vi "butterworth_comparison.vi"() -> ()   [LabVIEW 2022 SP3]
uses:
  <vilib>/express/express analysis/Spectral/Block/exnSpectralBlock spectral measurements peak poly.vi
  <vilib>/express/express analysis/Spectral/Block/exnSpectralBlock spectral measurements peak DDT.vi
  <vilib>/express/express analysis/Spectral/XNode/ExpressSpectralMeasurementsBlockNode.xnode
panel:
  out "Waveform Graph 4":dbl[][](graph)
  out "Waveform Graph 3":dbl[][](graph)
  out "Waveform Graph 2":dynamicdata(graph)
  out "Waveform Graph":dynamicdata(graph)
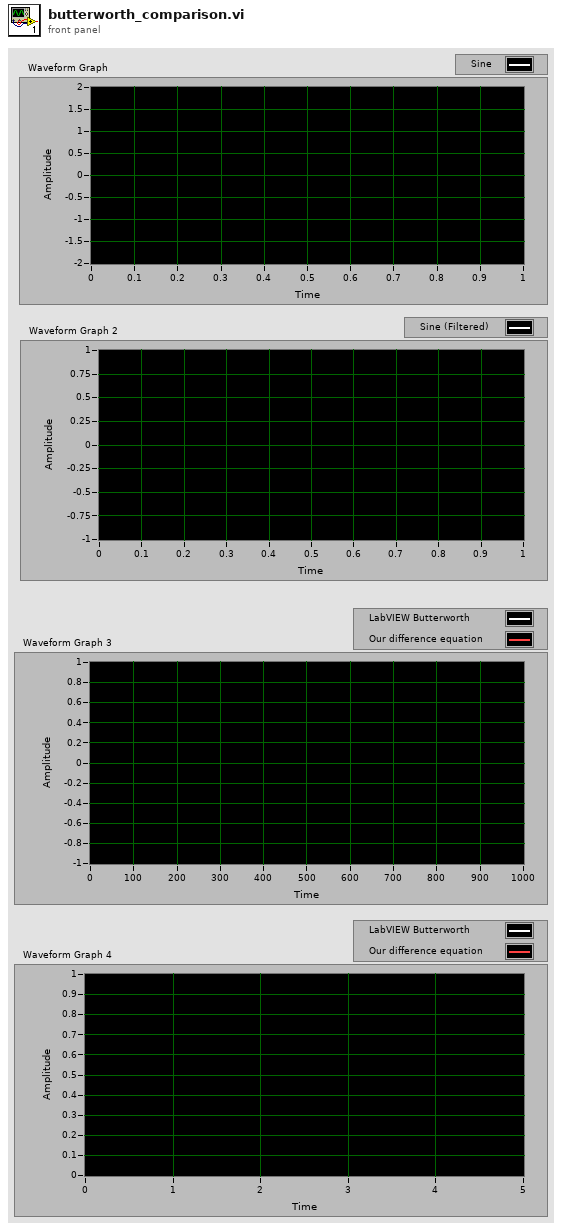
[diagram p1: front panel]
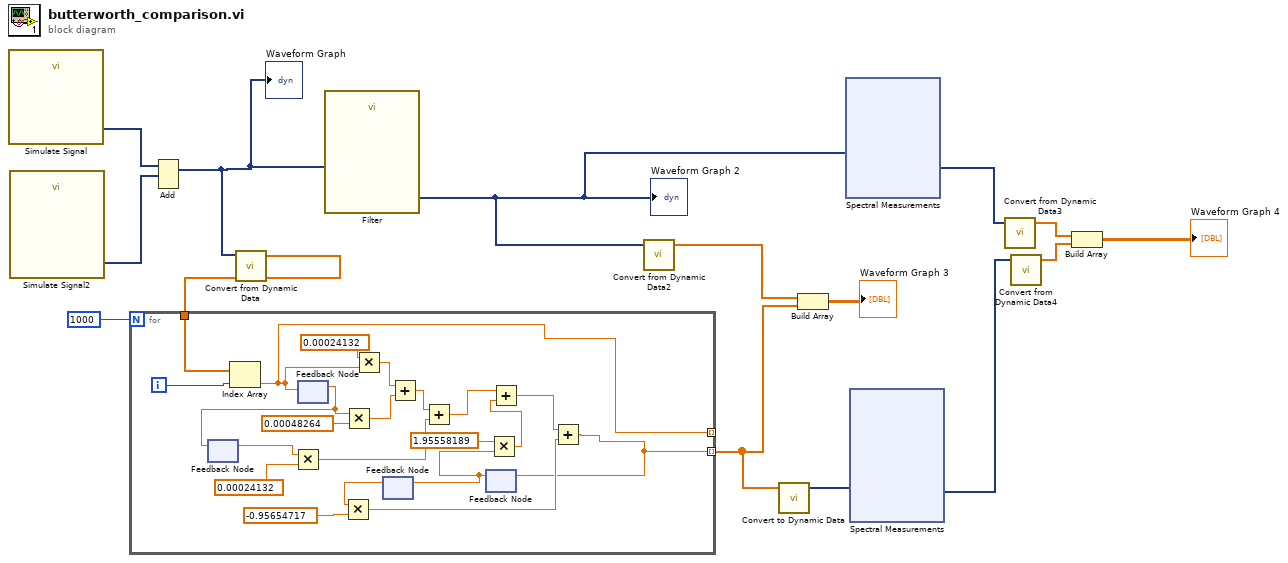
[diagram p0: block diagram]
diagram:
  n1 = call "Simulate Signal"() -> ("Sine"=w15:dynamicdata)  [unwired: 14 in, 1 out]
  n2 = call "Simulate Signal2"() -> ("Sine"=w14:dynamicdata)  [unwired: 14 in, 1 out]
  n3 = Add(1:w14, 2:w15) -> (0:w13:dynamicdata)  [unwired: 1 in, 1 out]
  "Waveform Graph" <- w13
  n4 = call "Convert from Dynamic Data"("Dynamic Data Type"=w13) -> ("Array"=w11:dbl[])  [unwired: 3 in]
  n5 = for {
    N: 1000 -> [_]
    tunnel: w11 -> [w30]
    tunnel: [w28] -> _ mode=indexing
    tunnel: [w16] -> w7 mode=indexing
    i -> [w29]
    n6 = feedback #1() -> (w23:dbl)  [unwired: 1 in]
    n7 = Index Array(array=w30, index=w29) -> (element=w28:dbl)
    n8 = Multiply(x=w23, y=0.00024132) -> (x*y=w20:dbl)
    n9 = feedback #2() -> (w24:dbl)  [unwired: 1 in]
    n10 = feedback-in #1(w24) -> ()
    n11 = feedback-in #2(w28) -> ()
    n12 = Multiply(x=w24, y=0.00048264) -> (x*y=w33:dbl)
    n13 = Multiply(x=0.00024132, y=w28) -> (x*y=w34:dbl)
    n14 = feedback #3() -> (w25:dbl)  [unwired: 1 in]
    n15 = Multiply(x=w25, y=-0.95654717) -> (x*y=w17:dbl)
    n16 = Add(x=w34, y=w33) -> (x+y=w21:dbl)
    n17 = Add(x=w21, y=w20) -> (x+y=w19:dbl)
    n18 = feedback #4() -> (w26:dbl)  [unwired: 1 in]
    n19 = feedback-in #3(w26) -> ()
    n20 = Multiply(x=1.95558189, y=w26) -> (x*y=w31:dbl)
    n21 = Add(x=w19, y=w31) -> (x+y=w18:dbl)
    n22 = Add(x=w18, y=w17) -> (x+y=w16:dbl)
    n23 = feedback-in #4(w16) -> ()
  }
  n24 = call "Filter"("Signal"=w13) -> ("Filtered Signal"=w8:dynamicdata)  [unwired: 9 in, 1 out]
  "Waveform Graph 2" <- w8
  n25 = call "Convert from Dynamic Data2"("Dynamic Data Type"=w8) -> ("Array"=w10:dbl[])  [unwired: 3 in]
  n26 = call "Convert to Dynamic Data"("Array"=w7) -> ("Dynamic Data Type"=w6:dynamicdata)  [unwired: 3 in]
  n27 = Build Array(w10, w7) -> (→"Waveform Graph 3":dbl[][])
  n28 = xnode "Spectral Measurements"("Signals"=w8) -> ("FFT - (Peak)"=w5:dynamicdata)  [unwired: 1 in, 2 out]
  n29 = xnode "Spectral Measurements"("Signals"=w6) -> ("FFT - (Peak)"=w4:dynamicdata)  [unwired: 1 in, 2 out]
  n30 = call "Convert from Dynamic Data3"("Dynamic Data Type"=w5) -> ("Array"=w3:dbl[])  [unwired: 3 in]
  n31 = call "Convert from Dynamic Data4"("Dynamic Data Type"=w4) -> ("Array"=w2:dbl[])  [unwired: 3 in]
  n32 = Build Array(w3, w2) -> (→"Waveform Graph 4":dbl[][])
